vi "drop.vi"(8 "error in (no error)":errorcluster, 10 "Regex":string) -> (0 "error out":errorcluster)   [LabVIEW 2015]
uses:
  C:/Users/Giuseppe/Downloads/LabLinda_ pakage/index_datatype.ctl
  C:/Users/Giuseppe/Downloads/LabLinda_ pakage/index_cluster.ctl
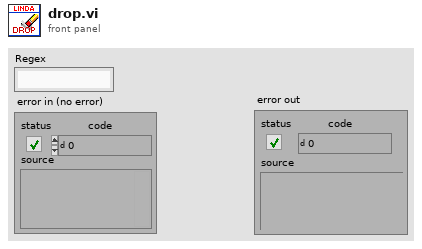
[diagram p1: front panel]
types:
  T1 = typedef "index_datatype.ctl" = T2[]
  T2 = typedef "index_cluster.ctl" = cluster{"Addr":i32[], "out react vi reference":refnum<vi>, "in react vi reference":refnum<vi>, "rd react vi reference":refnum<vi>, "Read_write_var":refnum<vi>}
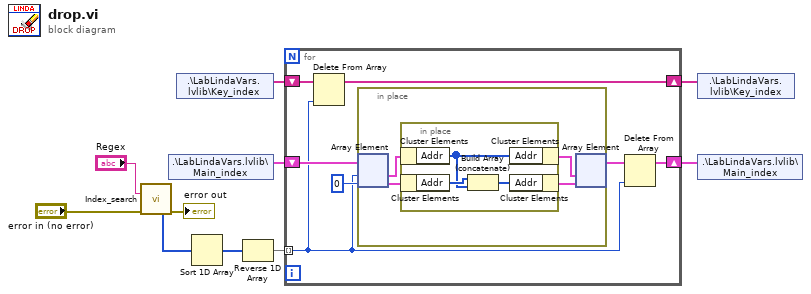
[diagram p0: block diagram]
diagram:
  n1 = call "Index_search.vi"("Regex"="Regex", "error in (no error)"="error in (no error)") -> ("Match index"=w5:i32[], "error out"=→"error out":errorcluster)  [unwired: 6 in, 6 out]
  n2 = shared-variable ".\\LabLindaVars.lvlib\\Main_index"() -> (w8:T1)  [unwired: 1 in, 1 out]
  n3 = shared-variable ".\\LabLindaVars.lvlib\\Key_index"() -> (w7:string[])  [unwired: 1 in, 1 out]
  n4 = Sort 1D Array(array=w5) -> (sorted array=w4:i32[])
  n5 = Reverse 1D Array(array=w4) -> (reversed array=w3:i32[])
  n6 = for {
    tunnel: w3 -> [w13] mode=indexing
    shift-right: [w12] -> w6
    shift-left: w8 -> [w17]
    shift-right: [w11] -> w1
    shift-left: w7 -> [w14]
    n7 = Delete From Array(array=w14, index=w13) -> (array with subset deleted=w11:string[])  [unwired: 1 in, 1 out]
    n8 = in-place {
      n9 = in-place-array #1(w17, w13, 0 ("index")) -> (w21:T2, w19:T2)
      n10 = in-place {
        n11 = in-place-cluster #2(w21) -> ("Addr"=w22:i32[])
        n12 = in-place-cluster #3(w19) -> ("Addr"=w23:i32[])
        n13 = Build Array (concatenate)(w23, w22) -> (w24:i32[])
        n14 = in-place-cluster #2("Addr"=w22) -> (w20:T2)
        n15 = in-place-cluster #3("Addr"=w24) -> (w18:T2)
      }
      n16 = in-place-array #1(w20, w18) -> (w15:T1)  [unwired: 2 out]
    }
    n17 = Delete From Array(array=w15, index=w13) -> (array with subset deleted=w12:T1)  [unwired: 1 in, 1 out]
  }
  n18 = shared-variable ".\\LabLindaVars.lvlib\\Key_index"(w1) -> ()  [unwired: 1 in, 1 out]
  n19 = shared-variable ".\\LabLindaVars.lvlib\\Main_index"(w6) -> ()  [unwired: 1 in, 1 out]
